vi "Write ConvBox.vi"(8 "error in":errorcluster, 9 "data":string, 10 "address string":string, 11 "VISA resource in":refnum<visa-resource-name>) -> (0 "error out":errorcluster, 2 "ibsta":T1, 3 "VISA resource out":refnum<visa-resource-name>)   [LabVIEW 2019, in "Localhost Protocols.lvlib" / "RS-xxx to GPIB ConvBox.lvclass"]
uses:
  RS-xxx to GPIB ConvBox.lvclass
  <vilib>/Instr/_visa.llb/GPIB Status Boolean Array.ctl
  <vilib>/Utility/error.llb/Clear Errors.vi
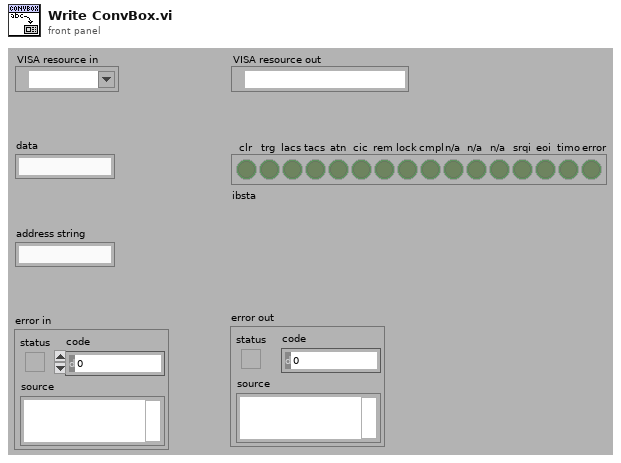
[diagram p1: front panel]
types:
  T1 = typedef "GPIB Status Boolean Array.ctl" = bool[]
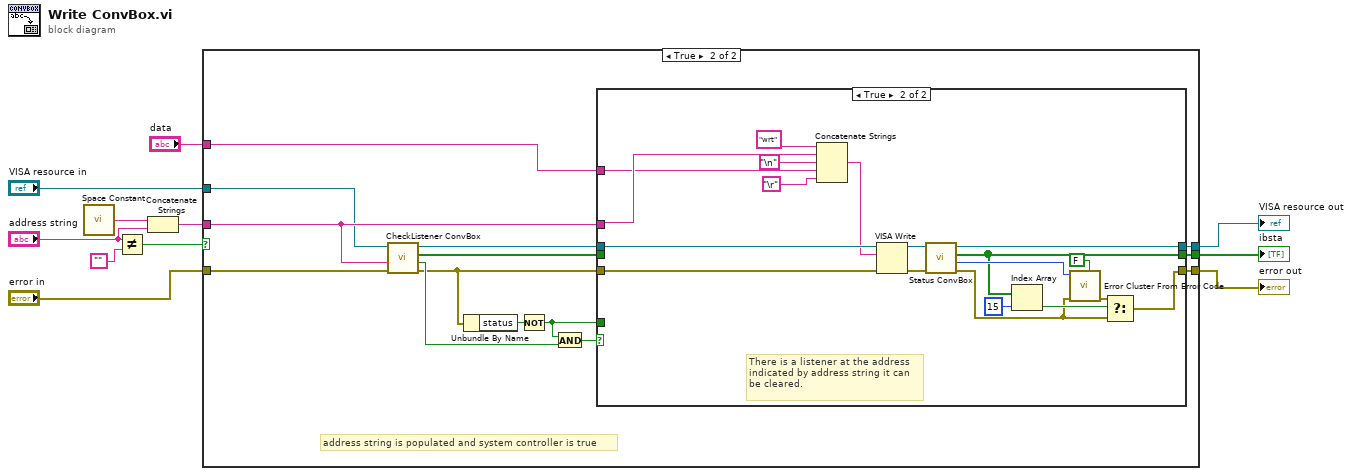
[diagram p0: block diagram]
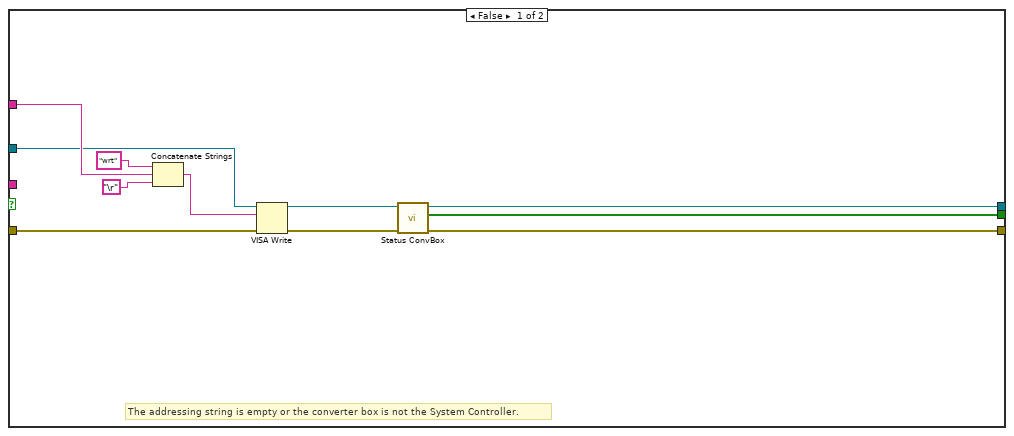
[diagram p2: hidden frame]
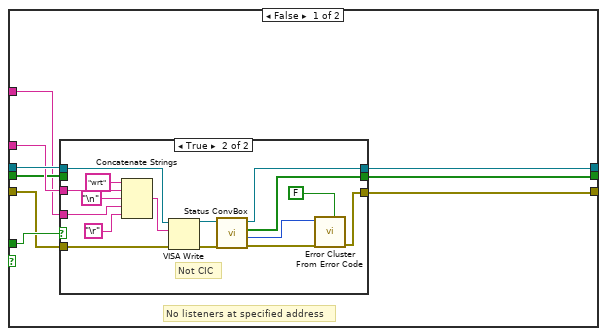
[diagram p3: hidden frame]
diagram:
  n1 = call <vilib>:"Space Constant.vi"() -> ("String"=w10:string)
  n2 = Not Equal?(x="address string", y="") -> (x != y?=w1:bool)
  n3 = Concatenate Strings(w10, "address string") -> (w9:string)
  n4 = case shown="True" w1 {
    tunnel: [w14 w36] -> w3
    tunnel: [w13 w35] -> w4
    tunnel: [w12 w34] -> w2
    tunnel: w9 -> [_ w31]
    tunnel: "error in" -> [w19 w33]
    tunnel: "VISA resource in" -> [w18 w30]
    tunnel: "data" -> [w21 w29]
    frame False {
      # "The addressing string is empty or the converter box is not the System Controller."
      n5 = Concatenate Strings("wrt", w21, "\r") -> (w17:string)
      n6 = VISA Write(VISA resource name=w18, write buffer=w17, error in (no error)=w19) -> (VISA resource name out=w15:refnum<visa-resource-name>, error out=w16:errorcluster)  [unwired: 1 out]
      n7 = call "Status ConvBox.vi"("error in (no error)"=w16, "VISA resource name"=w15) -> ("error out"=w12:errorcluster, "ibsta"=w13:T1, "VISA resource out"=w14:refnum<visa-resource-name>)  [unwired: 6 in, 1 out]
    }
    frame True {
      # "address string is populated and system controller is true"
      n8 = call "CheckListener ConvBox.vi"("error in"=w33, "address string"=w31, "VISA resource in"=w30) -> ("error out"=w26:errorcluster, "listener found"=w27:bool, "ibsta"=w23:T1, "VISA resource out"=w32:refnum<visa-resource-name>)  [unwired: 5 in]
      n9 = Unbundle By Name(w26) -> ("status"=w28:bool)
      n10 = Not(x=w28) -> (.not. x?=w24:bool)
      n11 = And(x=w24, y=w27) -> (x .and. y?=w25:bool)
      n12 = case shown="True" w25 {
        tunnel: [w39 w83] -> w36
        tunnel: [w40 w67] -> w35
        tunnel: [w38 w66] -> w34
        tunnel: w26 -> [w42 w80]
        tunnel: w32 -> [w45 w79]
        tunnel: w31 -> [w43 w76]
        tunnel: w29 -> [w37 w75]
        tunnel: w24 -> [w44 _]
        tunnel: w23 -> [w41 _]
        frame False {
          # "No listeners at specified address"
          n13 = case shown="True" w44 {
            tunnel: [w46 w63] -> w38
            tunnel: w42 -> [w46 w62]
            tunnel: w45 -> [w47 w58]
            tunnel: [w47 w57] -> w39
            tunnel: [w48 w55] -> w40
            tunnel: w43 -> [_ w49]
            tunnel: w41 -> [w48 _]
            tunnel: w37 -> [_ w50]
            frame False {
            }
            frame True {
              # "Not CIC"
              n14 = Concatenate Strings("wrt", w49, "\n", w50, "\r") -> (w51:string)
              n15 = VISA Write(VISA resource name=w58, write buffer=w51, error in (no error)=w62) -> (VISA resource name out=w59:refnum<visa-resource-name>, error out=w61:errorcluster)  [unwired: 1 out]
              n16 = call "Status ConvBox.vi"("error in (no error)"=w61, "VISA resource name"=w59) -> ("error out"=w60:errorcluster, "GPIB error"=w56:i16, "ibsta"=w55:T1, "VISA resource out"=w57:refnum<visa-resource-name>)  [unwired: 6 in]
              n17 = call <vilib>:"Error Cluster From Error Code.vi"("is warning? (False)"=FALSE, "error in (no error)"=w60, "error code (0)"=w56) -> ("error out"=w63:errorcluster)  [unwired: 6 in]
            }
          }
        }
        frame True {
          # "There is a listener at the address\nindicated by address string it can\nbe cleared."
          n18 = Concatenate Strings("wrt", w76, "\n", w75, "\r") -> (w74:string)
          n19 = VISA Write(VISA resource name=w79, write buffer=w74, error in (no error)=w80) -> (VISA resource name out=w82:refnum<visa-resource-name>, error out=w81:errorcluster)  [unwired: 1 out]
          n20 = call "Status ConvBox.vi"("error in (no error)"=w81, "VISA resource name"=w82) -> ("error out"=w69:errorcluster, "GPIB error"=w68:i16, "ibsta"=w67:T1, "VISA resource out"=w83:refnum<visa-resource-name>)  [unwired: 6 in]
          n21 = Index Array(array=w67, index=15) -> (element=w71:bool)
          n22 = call <vilib>:"Error Cluster From Error Code.vi"("is warning? (False)"=FALSE, "error in (no error)"=w69, "error code (0)"=w68) -> ("error out"=w70:errorcluster)  [unwired: 6 in]
          n23 = Select(t=w70, s=w71, f=w69) -> (s? t:f=w66:errorcluster)
        }
      }
    }
  }
  "VISA resource out" <- w3
  "error out" <- w2
  "ibsta" <- w4
